vi "Clousure.vi"(8 "error in (no error)":errorcluster, 11 "ConcreteProductB in":refnum<class "ConcreteProductB.lvclass">) -> (0 "error out":errorcluster, 3 "ConcreteProductB out":refnum<class "ConcreteProductB.lvclass">)   [LabVIEW 2020, in "FactoryMethod.lvlib" / "ConcreteProductB.lvclass"]
uses:
  ConcreteProductB.lvclass
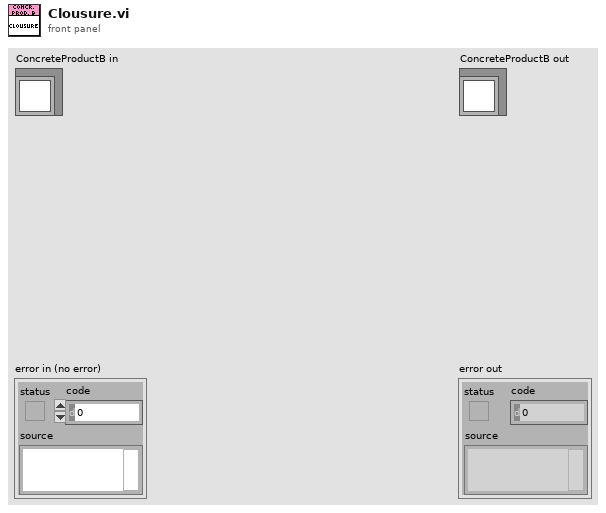
[diagram p1: front panel]
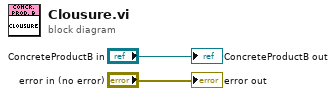
[diagram p0: block diagram]
diagram:
  "error out" <- "error in (no error)"
  "ConcreteProductB out" <- "ConcreteProductB in"
